vi "Connect.vi"(6 "deadline":T1={"mode"=enum."Relative", "deadline (ms)"=30000}, 8 "error in":errorcluster, 9 "user@host":string, 10 "client in":refnum<class "Generic Client.lvclass">, 11 "connection in":refnum<class "Low Level Connection.lvclass">) -> (0 "error out":errorcluster, 2 "session out":refnum<class "Generic Client.lvclass">, 3 "connection out":refnum<class "Low Level Connection.lvclass">)   [LabVIEW 2020, in "NI_SFTP.lvlib" / "Low Level Connection.lvclass"]
doc: "Connect to an SFTP server."
uses:
  <vilib>/net/SFTP/Low Level Connection/Low Level Connection.lvclass
  <vilib>/net/SSH/Client/Generic/Generic Client.lvclass
  <vilib>/Utility/Deadline/Deadline.ctl
  <vilib>/Utility/Deadline/Mode.ctl
  <vilib>/Utility/Deadline/NI_Deadline.lvlib
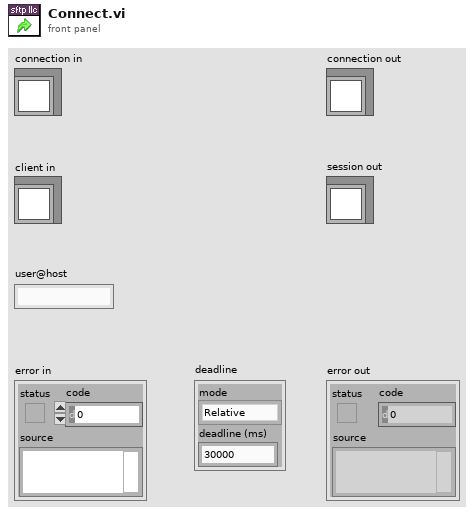
[diagram p1: front panel]
types:
  T1 = typedef "NI_Deadline.lvlib/Deadline.ctl" = cluster{"mode":T2, "deadline (ms)":u32}
  T2 = typedef "NI_Deadline.lvlib/Mode.ctl" = enum16{"Relative", "Use deadline", "Wait forever", "Nonblocking", "N/A"}
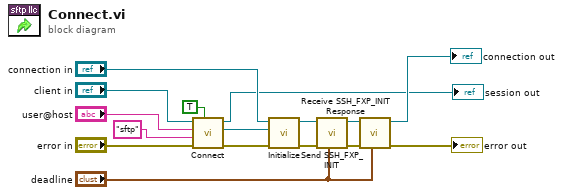
[diagram p0: block diagram]
diagram:
  n1 = call-dynamic "Connect.vi"("command is subsystem"=TRUE ("subsystem?"), "error in (no error)"="error in", "command"="sftp" ("subsystem"), "user@host"="user@host", "session in"="client in") -> ("error out"=w15:errorcluster, "SSH subprocess"=w5:refnum<class "Subprocess.lvclass">, "session out"=→"session out":refnum<class "Generic Client.lvclass">)  [unwired: 4 in]
  n2 = call <vilib>:"Initialize.vi"("error in"=w15, "client in"=w5, "connection in"="connection in") -> ("error out"=w12:errorcluster, "connection out"=w13:refnum<class "Low Level Connection.lvclass">)  [unwired: 7 in]
  n3 = call <vilib>:"Send SSH_FXP_INIT.vi"("deadline"="deadline", "error in"=w12, "connection in"=w13) -> ("error out"=w10:errorcluster, "connection out"=w11:refnum<class "Low Level Connection.lvclass">)  [unwired: 7 in]
  n4 = call <vilib>:"Receive SSH_FXP_INIT Response.vi"("deadline"="deadline", "error in"=w10, "connection in"=w11) -> ("error out"=→"error out":errorcluster, "connection out"=→"connection out":refnum<class "Low Level Connection.lvclass">)  [unwired: 7 in]
